vi "Write Z speed.vi"(8 "error in (no error)":errorcluster, 10 "Z speed":dbl, 11 "Dispense in":refnum<class "Dispense.lvclass">) -> (0 "error out":errorcluster, 3 "Dispense out":refnum<class "Dispense.lvclass">)   [LabVIEW 2020, in "Dispense.lvclass"]
uses:
  Dispense.lvclass
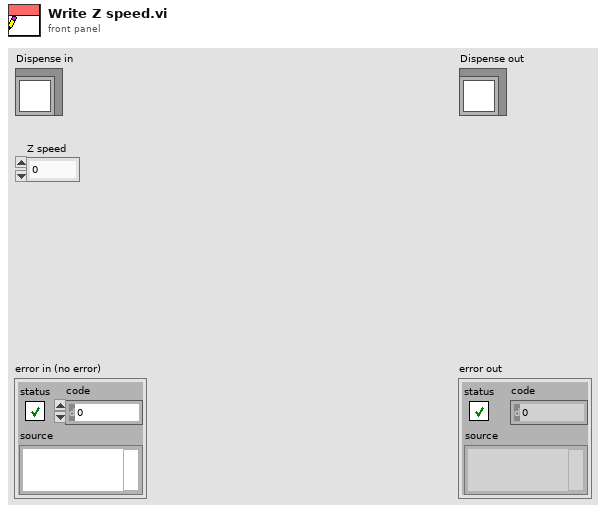
[diagram p1: front panel]
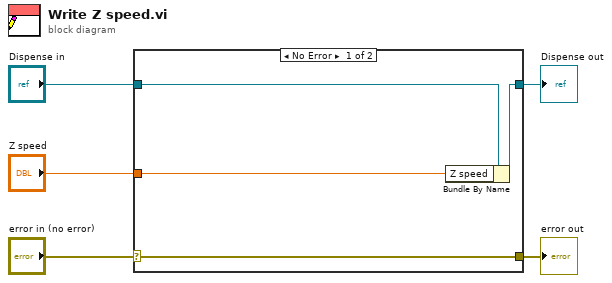
[diagram p0: block diagram]
diagram:
  n1 = case shown="No Error" "error in (no error)" {
    selector: "error in (no error)" -> [w9 w10]
    tunnel: [w9 w10] -> w4
    tunnel: [w7 w11] -> w2
    tunnel: "Dispense in" -> [w8 w11]
    tunnel: "Z speed" -> [w6 _]
    frame No Error {
      n2 = Bundle By Name(cluster=w8, "Z speed"=w6) -> (w7:refnum<class "Dispense.lvclass">)
    }
    frame Error {
    }
  }
  "error out" <- w4
  "Dispense out" <- w2
